vi "OP20 Indicators.vi"(8 "error in (no error)":errorcluster, 10 "Array":refnum<vi>[](array[refnum]), 11 "OUTPUT INDICATOR":T1={"OP - 10"={"BARCODE"="", "LEAK RATE"=0.0, "RESULT"=FALSE}, "OP - 30"={"BARCODE"="", "Displacement"=0.0, "Load"=0.0, "Middle Gear Shaft Status"=FALSE, "Final Result"=FALSE}, "OP - 60"={"BARCODE"="", "Screw 1 Data"=0.0, "Screw 2 data"=0.0, "Screw 1 Status"=FALSE, "Screw 2 Status"=FALSE, "Screw3 Data"=0.0, "Final Result"=FALSE, "Screw3 Status"=FALSE, "Screw4 Data"=0.0, "Screw5 Data"=0.0, "Screw4 Status"=FALSE, "Screw5 Status"=FALSE, "Screw6 Data"=0.0, "Screw6 Status"=FALSE}, "OP - 70"={"BARCODE"="", "Sensor MIN Vltg"=0.0, "Sensor MAX Vltg"=0.0, "Final Result"=FALSE}, "OP - 80"={"BARCODE"="", "Load"=0.0, "Final Result"=FALSE, "Dispensing"=FALSE}, "OP - 90"={"BARCODE"="", "Seat LT Data"=0.0, "Seat Status"=FALSE, "Steam LT Data"=0.0, "Final Result"=FALSE}, "OP - 110"={"BARCODE"=""}, "OP - 20"={"BARCODE"="", "Bottom Displace"=0.0, "Bottom Load"=0.0, "Camera Status"=FALSE, "Bottom Result"=TRUE, "Top Displace"=0.0, "Top Load "=0.0, "Camera Status"=FALSE, "Top Result"=FALSE, "Final Result"=FALSE}, "OP - 50"={"BARCODE"="", "Nut Torque"=0.0, "LH Motor Screw"=0.0, "LH Status"=FALSE, "RH Status"=FALSE, "RH Motor Screw"=0.0, "Final Result"=FALSE, "Nut Status"=FALSE, "Camera Status"=FALSE}, "OP - 100"={"BARCODE"="", "Sensor O/P Open"=0.0, "Sensor O/P Start Of Close"=0.0, "Final Result"=FALSE, "Sensor O/P Full Close"=0.0, "Motor Peak"=0.0, "Motor Start Of Close"=0.0, "Motor Full Close"=0.0, "Motor Start Back"=0.0, "Motor Full Open"=0.0, "Response time FWD"=0.0, "Response Time REV"=0.0, "Camera Status"=FALSE}, "OP - 40"={"BARCODE"="", "RH Screw"=0.0, "LH Screw "=0.0, "RH Status"=FALSE, "LH Status"=FALSE, "Dispalcement "=0.0, "Stack Load "=0.0, "Final Result"=FALSE, "Camera Status"=TRUE}}) -> (0 "error out":errorcluster, 3 "OUTPUT INDICATOR":T1={"OP - 10"={"BARCODE"="", "LEAK RATE"=0.0, "RESULT"=FALSE}, "OP - 30"={"BARCODE"="", "Displacement"=0.0, "Load"=0.0, "Middle Gear Shaft Status"=FALSE, "Final Result"=FALSE}, "OP - 60"={"BARCODE"="", "Screw 1 Data"=0.0, "Screw 2 data"=0.0, "Screw 1 Status"=FALSE, "Screw 2 Status"=FALSE, "Screw3 Data"=0.0, "Final Result"=FALSE, "Screw3 Status"=FALSE, "Screw4 Data"=0.0, "Screw5 Data"=0.0, "Screw4 Status"=FALSE, "Screw5 Status"=FALSE, "Screw6 Data"=0.0, "Screw6 Status"=FALSE}, "OP - 70"={"BARCODE"="", "Sensor MIN Vltg"=0.0, "Sensor MAX Vltg"=0.0, "Final Result"=FALSE}, "OP - 80"={"BARCODE"="", "Load"=0.0, "Final Result"=FALSE, "Dispensing"=FALSE}, "OP - 90"={"BARCODE"="", "Seat LT Data"=0.0, "Seat Status"=FALSE, "Steam LT Data"=0.0, "Final Result"=FALSE}, "OP - 110"={"BARCODE"=""}, "OP - 20"={"BARCODE"="", "Bottom Displace"=0.0, "Bottom Load"=0.0, "Camera Status"=FALSE, "Bottom Result"=TRUE, "Top Displace"=0.0, "Top Load "=0.0, "Camera Status"=FALSE, "Top Result"=FALSE, "Final Result"=FALSE}, "OP - 50"={"BARCODE"="", "Nut Torque"=0.0, "LH Motor Screw"=0.0, "LH Status"=FALSE, "RH Status"=FALSE, "RH Motor Screw"=0.0, "Final Result"=FALSE, "Nut Status"=FALSE, "Camera Status"=FALSE}, "OP - 100"={"BARCODE"="", "Sensor O/P Open"=0.0, "Sensor O/P Start Of Close"=0.0, "Final Result"=FALSE, "Sensor O/P Full Close"=0.0, "Motor Peak"=0.0, "Motor Start Of Close"=0.0, "Motor Full Close"=0.0, "Motor Start Back"=0.0, "Motor Full Open"=0.0, "Response time FWD"=0.0, "Response Time REV"=0.0, "Camera Status"=FALSE}, "OP - 40"={"BARCODE"="", "RH Screw"=0.0, "LH Screw "=0.0, "RH Status"=FALSE, "LH Status"=FALSE, "Dispalcement "=0.0, "Stack Load "=0.0, "Final Result"=FALSE, "Camera Status"=TRUE}})   [LabVIEW 2017]
uses:
  Control/OUTPUT Cluster Indicator.ctl
  8bcb6a2e-dfd2-4f6b-b5e2-eb446c823387.vi
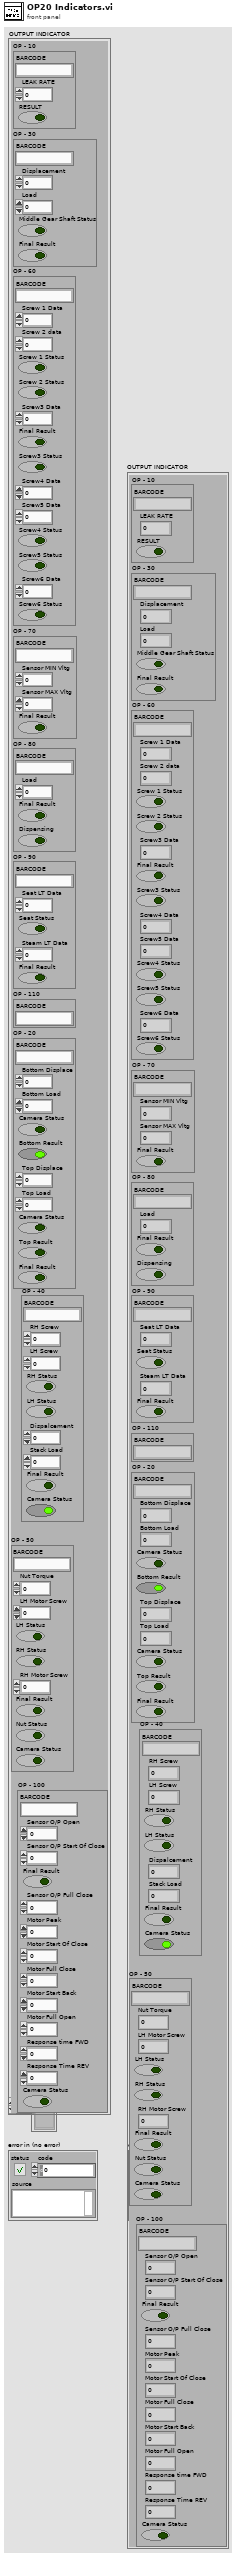
[diagram p1: front panel]
types:
  T1 = typedef "OUTPUT Cluster Indicator.ctl" = cluster{"OP - 10":cluster{"BARCODE":string, "LEAK RATE":dbl, "RESULT":bool}, "OP - 30":cluster{"BARCODE":string, "Displacement":dbl, "Load":dbl, "Middle Gear Shaft Status":bool, "Final Result":bool}, "OP - 60":cluster{"BARCODE":string, "Screw 1 Data":dbl, "Screw 2 data":dbl, "Screw 1 Status":bool, "Screw 2 Status":bool, "Screw3 Data":dbl, "Final Result":bool, "Screw3 Status":bool, "Screw4 Data":dbl, "Screw5 Data":dbl, "Screw4 Status":bool, "Screw5 Status":bool, "Screw6 Data":dbl, "Screw6 Status":bool}, "OP - 70":cluster{"BARCODE":string, "Sensor MIN Vltg":dbl, "Sensor MAX Vltg":dbl, "Final Result":bool}, "OP - 80":cluster{"BARCODE":string, "Load":dbl, "Final Result":bool, "Dispensing":bool}, "OP - 90":cluster{"BARCODE":string, "Seat LT Data":dbl, "Seat Status":bool, "Steam LT Data":dbl, "Final Result":bool}, "OP - 110":cluster{"BARCODE":string}, "OP - 20":cluster{"BARCODE":string, "Bottom Displace":dbl, "Bottom Load":dbl, "Camera Status":bool, "Bottom Result":bool, "Top Displace":dbl, "Top Load ":dbl, "Camera Status":bool, "Top Result":bool, "Final Result":bool}, "OP - 50":cluster{"BARCODE":string, "Nut Torque":dbl, "LH Motor Screw":dbl, "LH Status":bool, "RH Status":bool, "RH Motor Screw":dbl, "Final Result":bool, "Nut Status":bool, "Camera Status":bool}, "OP - 100":cluster{"BARCODE":string, "Sensor O/P Open":dbl, "Sensor O/P Start Of Close":dbl, "Final Result":bool, "Sensor O/P Full Close":dbl, "Motor Peak":dbl, "Motor Start Of Close":dbl, "Motor Full Close":dbl, "Motor Start Back":dbl, "Motor Full Open":dbl, "Response time FWD":dbl, "Response Time REV":dbl, "Camera Status":bool}, "OP - 40":cluster{"BARCODE":string, "RH Screw":dbl, "LH Screw ":dbl, "RH Status":bool, "LH Status":bool, "Dispalcement ":dbl, "Stack Load ":dbl, "Final Result":bool, "Camera Status":bool}}
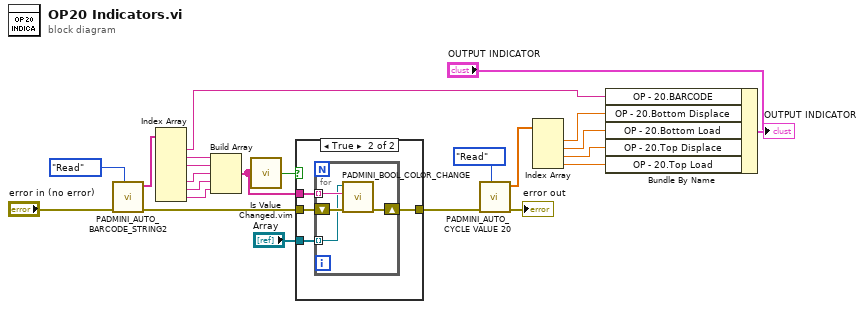
[diagram p0: block diagram]
diagram:
  n1 = call "PADMINI_AUTO_BARCODE_STRING2.vi"("Enum"=enum16{"Read", "Write"}."Read", "error in (no error)"="error in (no error)") -> ("error out"=w5:errorcluster, "Input 2"=w4:string[])  [unwired: 8 in]
  n2 = Index Array(array=w4) -> (element #1=w2:string, element #2=w13:string, element #3=w14:string, element #5=w15:string, element #6=w16:string, element #7=w17:string)  [unwired: 7 in, 1 out]
  n3 = Build Array(w13, w14, w15, w16, w17) -> (w18:string[])
  n4 = call "Is Value Changed.vim"("value"=w18) -> ("changed or first call?"=w1:bool)
  n5 = case shown="True" w1 {
    tunnel: [w24 w28] -> w21
    tunnel: w18 -> [_ w27]
    tunnel: w5 -> [w24 w26]
    tunnel: "Array" -> [_ w25]
    frame False {
    }
    frame True {
      n6 = for {
        tunnel: w27 -> [w31] mode=indexing
        shift-right: [w32] -> w28
        shift-left: w26 -> [w30]
        tunnel: w25 -> [w29] mode=indexing
        n7 = call "PADMINI_BOOL_COLOR_CHANGE.vi"("error in (no error)"=w30, "Input Result"=w31, "Boolean in"=w29) -> ("error out"=w32:errorcluster)  [unwired: 8 in]
      }
    }
  }
  n8 = call "PADMINI_AUTO_CYCLE VALUE 20.vi"("Enum"=enum16{"Read", "Write"}."Read", "error in (no error)"=w21) -> ("error out"=→"error out":errorcluster, "Input 2"=w20:sgl[])  [unwired: 8 in]
  n9 = Index Array(array=w20) -> (element #1=w6:sgl, element #2=w9:sgl, element #3=w10:sgl, element #4=w11:sgl)  [unwired: 4 in]
  n10 = Bundle By Name(cluster="OUTPUT INDICATOR", "OP - 20.BARCODE"=w2, "OP - 20.Bottom Displace"=w6, "OP - 20.Bottom Load"=w9, "OP - 20.Top Displace"=w10, "OP - 20.Top Load"=w11) -> (→"OUTPUT INDICATOR":T1)
